vi "decide_type.vi"(10 "Class Hierarchy":string[](array[string]), 11 "OriginalClassname":string) -> (3 "OutputType":string)   [LabVIEW 2020]
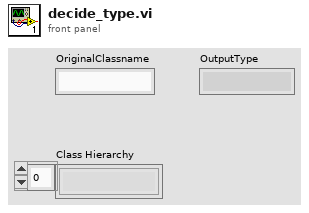
[diagram p1: front panel]
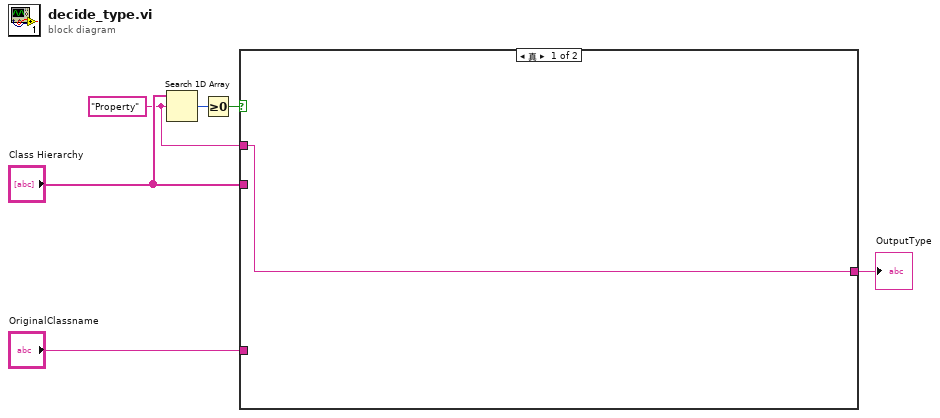
[diagram p0: block diagram]
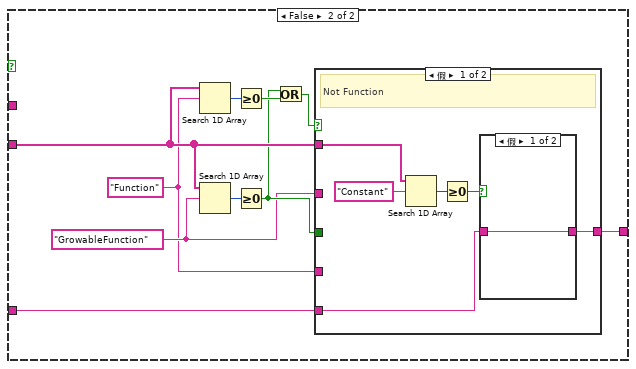
[diagram p2: hidden frame]
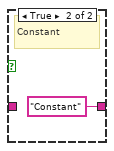
[diagram p3: hidden frame]
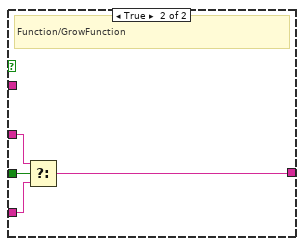
[diagram p4: hidden frame]
diagram:
  w1 = "Property" ("元素")
  n1 = Search 1D Array ("搜索一维数组")(1D array="Class Hierarchy", element=w1) -> (index of element=w4:i32)  [unwired: 1 in]
  n2 = Greater Or Equal To 0? ("大于等于0？")(x=w4) -> (x >= 0?=w2:bool)
  n3 = case shown="真" w2 {
    tunnel: [w7 w13] -> w6
    tunnel: "Class Hierarchy" -> [_ w12]
    tunnel: "OriginalClassname" -> [_ w8]
    tunnel: w1 -> [w7 _]
    frame True {
    }
    frame False {
      w9 = "Function" ("元素")
      w10 = "GrowableFunction" ("元素")
      n4 = Search 1D Array ("搜索一维数组")(1D array=w12, element=w9) -> (index of element=w16:i32)  [unwired: 1 in]
      n5 = Search 1D Array ("搜索一维数组")(1D array=w12, element=w10) -> (index of element=w17:i32)  [unwired: 1 in]
      n6 = Greater Or Equal To 0? ("大于等于0？")(x=w16) -> (x >= 0?=w15:bool)
      n7 = Greater Or Equal To 0? ("大于等于0？")(x=w17) -> (x >= 0?=w11:bool)
      n8 = Or ("或")(x=w11, y=w15) -> (x .or. y?=w14:bool)
      n9 = case shown="假" w14 {
        tunnel: [w19 w26] -> w13
        tunnel: w12 -> [w21 _]
        tunnel: w8 -> [w18 _]
        tunnel: w11 -> [_ w28]
        tunnel: w10 -> [_ w29]
        tunnel: w9 -> [_ w27]
        frame False {
          # "Not Function"
          n10 = Search 1D Array ("搜索一维数组")(1D array=w21, element="Constant" ("元素")) -> (index of element=w23:i32)  [unwired: 1 in]
          n11 = Greater Or Equal To 0? ("大于等于0？")(x=w23) -> (x >= 0?=w20:bool)
          n12 = case shown="假" w20 {
            tunnel: [w24 "Constant" ("元素")] -> w19
            tunnel: w18 -> [w24 _]
            frame False {
            }
            frame True {
              # "Constant"
            }
          }
        }
        frame True {
          # "Function/GrowFunction"
          n13 = Select ("选择")(t=w29, s=w28, f=w27) -> (s? t:f=w26:string)
        }
      }
    }
  }
  "OutputType" <- w6
